vi "Create Custom Char.vi"(7 "Char #":u8, 8 "error in (no error)":errorcluster, 9 "Char":T1=[[FALSE, FALSE, FALSE, FALSE, FALSE], [FALSE, FALSE, FALSE, FALSE, FALSE], [FALSE, FALSE, FALSE, FALSE, FALSE], [FALSE, FALSE, FALSE, FALSE, FALSE], [FALSE, FALSE, FALSE, FALSE, FALSE], [FALSE, FALSE, FALSE, FALSE, FALSE], [FALSE, FALSE, FALSE, FALSE, FALSE], [FALSE, FALSE, FALSE, FALSE, FALSE]], 11 "Character LCD in":refnum<class "Char LCD.lvclass">) -> (0 "error out":errorcluster, 3 "Character LCD out":refnum<class "Char LCD.lvclass">)   [LabVIEW 2020, in "CTI-Peripheral.lvlib" / "Char LCD.lvclass"]
uses:
  Char LCD.lvclass
  Custom Char.ctl
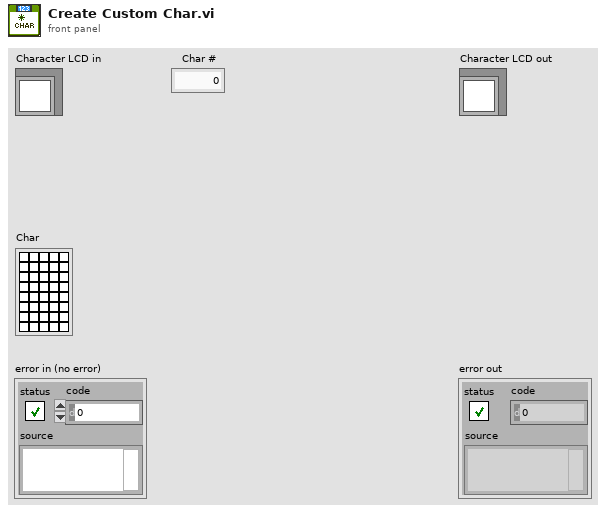
[diagram p1: front panel]
types:
  T1 = typedef "CTI-Peripheral.lvlib/Char LCD.lvclass/Custom Char.ctl" = bool[][]
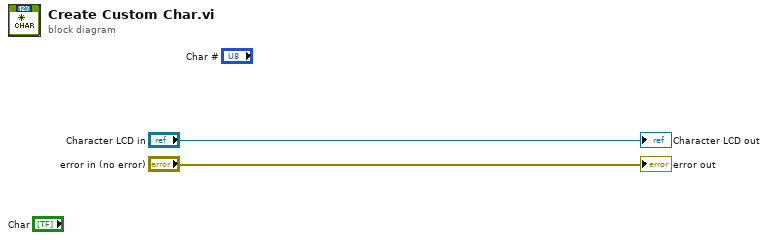
[diagram p0: block diagram]
diagram:
  "error out" <- "error in (no error)"
  "Character LCD out" <- "Character LCD in"
